vi "Port Number and Machine Name.vi"(0 "LV RT in":refnum<class "LV RT.lvclass">, 5 "PID":string, 11 "error in (no error)":errorcluster) -> (4 "LV RT out":refnum<class "LV RT.lvclass">, 6 "Machine Name":string, 8 "Port Number":u16, 15 "error out":errorcluster)   [LabVIEW 2016, in "LV RT.lvclass"]
uses:
  LV RT.lvclass
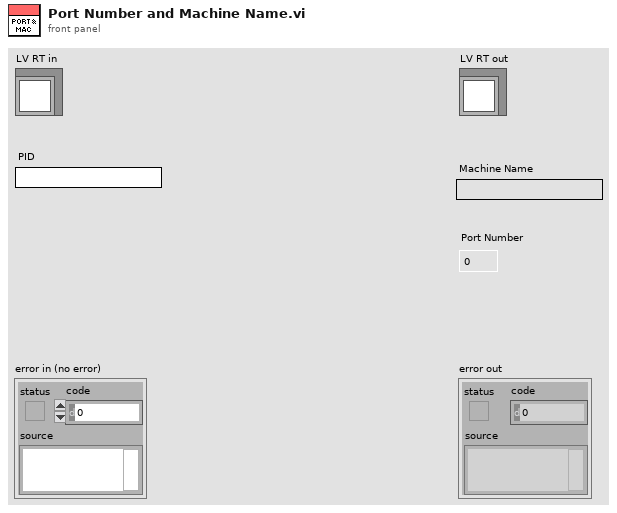
[diagram p1: front panel]
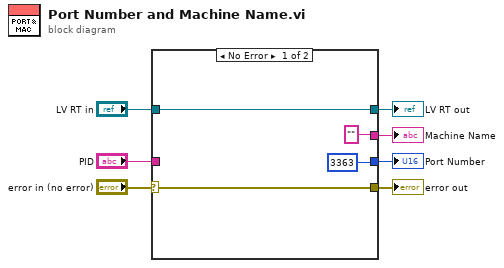
[diagram p0: block diagram]
diagram:
  n1 = case shown="No Error" "error in (no error)" {
    selector: "error in (no error)" -> [w11 w13]
    tunnel: [w11 w13] -> w6
    tunnel: "LV RT in" -> [w10 w12]
    tunnel: [w10 w12] -> w4
    tunnel: ["" _] -> w3
    tunnel: [u16 3363 _] -> w2
    tunnel: "PID" -> [_ _]
    frame No Error {
    }
    frame Error {
    }
  }
  "error out" <- w6
  "LV RT out" <- w4
  "Port Number" <- w2
  "Machine Name" <- w3
